vi "EF_GetFeaturesVectorEntropy.vi"(8 "error in (no error)":errorcluster, 9 "Amplitude Min":dbl, 10 "Amplitude Max":dbl, 11 "Array Of Waveforms in":waveform(dbl)[](array[waveform])) -> (0 "error out":errorcluster, 3 "Features Array out":dbl[][](array[numeric]))   [LabVIEW 2016, in "Feature Extraction.lvlib"]
uses:
  Feature Extraction.lvlib
panel:
  # "This VI is a part of BCI Design library, http://www.ru-bci.org \nCopyright © 2020, Sotnikov Peter, All rights reserved. License: GNU GPLv3"
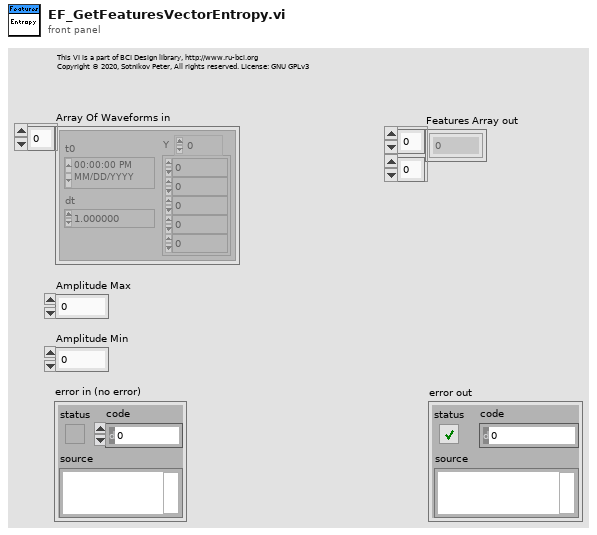
[diagram p1: front panel]
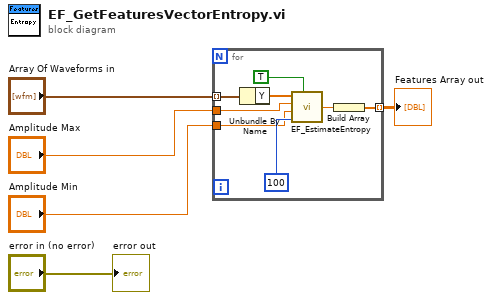
[diagram p0: block diagram]
diagram:
  n1 = for {
    tunnel: "Array Of Waveforms in" -> [w13] mode=indexing
    tunnel: [w10] -> w4 mode=indexing
    tunnel: "Amplitude Max" -> [w7]
    tunnel: "Amplitude Min" -> [w6]
    n2 = Unbundle By Name(w13) -> ("Y"=w9:dbl[])
    n3 = call "EF_EstimateEntropy.vi"("Array in"=w9, "X max"=w7, "X min"=w6, "# bins"=100, "Normalized ?"=TRUE) -> ("Shannon Entropy out"=w12:dbl)
    n4 = Build Array(w12) -> (w10:dbl[])
  }
  "Features Array out" <- w4
  "error out" <- "error in (no error)"
